vi "Sagar C V 4 X 1 Multiplexer (1).vi"() -> ()   [LabVIEW 2018]
panel:
  out "Y":bool
  in  "S0":bool
  in  "S1":bool
  in  "I3":bool
  in  "I2":bool
  in  "I1":bool
  in  "I0":bool
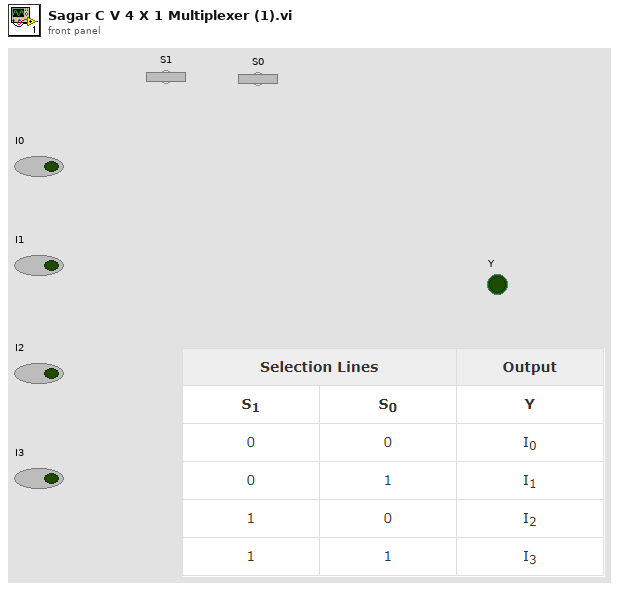
[diagram p1: front panel]
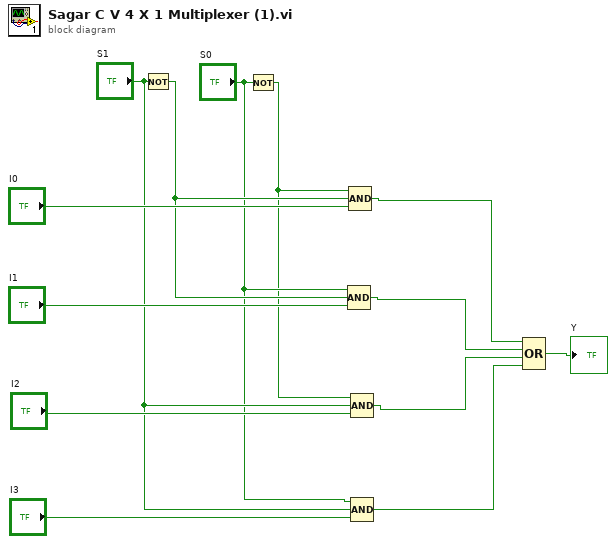
[diagram p0: block diagram]
diagram:
  n1 = Not(x="S1") -> (.not. x?=w8:bool)
  n2 = Not(x="S0") -> (.not. x?=w6:bool)
  n3 = Compound Arithmetic op=AND("S0", w8, "I1") -> (w4:bool)
  n4 = Compound Arithmetic op=AND(w6, w8, "I0") -> (w5:bool)
  n5 = Compound Arithmetic op=AND(w6, "S1", "I2") -> (w3:bool)
  n6 = Compound Arithmetic op=AND("S0", "S1", "I3") -> (w2:bool)
  n7 = Compound Arithmetic op=OR(w5, w4, w3, w2) -> (→"Y":bool)
